vi "YAML Parser Errors Code Offset.vi"() -> (0 "YAML Parser Errors Code Offset":i32)   [LabVIEW 2015, in "YAML Parser.lvlib"]
uses:
  YAML Parser.lvlib
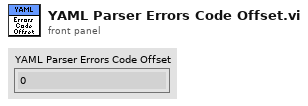
[diagram p1: front panel]
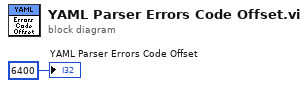
[diagram p0: block diagram]
diagram:
  "YAML Parser Errors Code Offset" <- 6400
